vi "clean ring control.vi"(8 "error in (no error)":errorcluster, 11 "Ring Ref":refnum<vi>[](array[refnum])) -> (0 "error out":errorcluster)   [LabVIEW 2024, in "Ring Control Management.lvlib"]
doc: "This VI removes all items from the Ring controls referenced in the <b>Ring Ref</b> array, leaving them empty with no items in their lists."
uses:
  Ring Control Management.lvlib
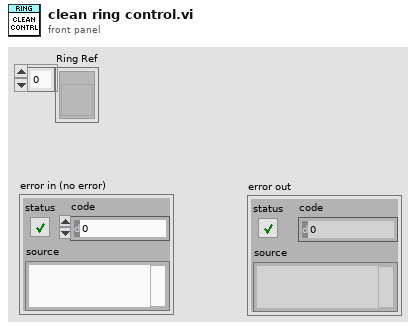
[diagram p1: front panel]
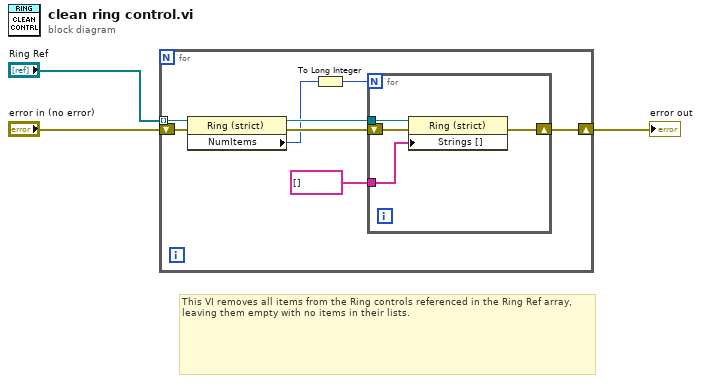
[diagram p0: block diagram]
diagram:
  # "This VI removes all items from the Ring controls referenced in the Ring Ref array, leaving them empty with no items in their lists."
  n1 = for {
    tunnel: "Ring Ref" -> [w10] mode=indexing
    shift-right: [w11] -> w3
    shift-left: "error in (no error)" -> [w5]
    n2 = property on="Property Node" class="Ring (strict)"(reference=w10, error in=w5) -> (reference out=w9:refnum<vi>, error out=w8:errorcluster, "NumItems"=w7:u32)
    n3 = To Long Integer(number=w7) -> (32bit integer=w4:i32)
    n4 = for {
      N: w4 -> [_]
      tunnel: w9 -> [w14]
      tunnel: string[] [] -> [w12]
      shift-right: [w15] -> w11
      shift-left: w8 -> [w13]
      n5 = property on="Property Node" class="Ring (strict)"(reference=w14, error in=w13, "Strings []"=w12) -> (error out=w15:errorcluster)  [unwired: 1 out]
    }
  }
  "error out" <- w3
